vi "RichToFlatmeasurement_StreamRequest.vi"(5 "OutputClusterType":T1, 11 "InputCluster":T2) -> (3 "OutputCluster":T1)   [LabVIEW 2021, in "Measurement_server.lvlib"]
uses:
  Measurement_server.lvlib
  measurement_StreamRequest.ctl
  measurement_StreamRequest_Flat.ctl
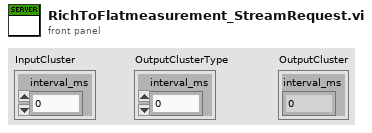
[diagram p1: front panel]
types:
  T1 = typedef "Measurement_server.lvlib/measurement_StreamRequest_Flat.ctl" = cluster{"interval_ms":i32}
  T2 = typedef "Measurement_server.lvlib/measurement_StreamRequest.ctl" = cluster{"interval_ms":i32}
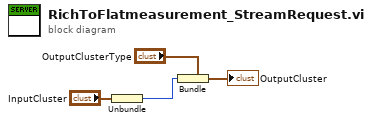
[diagram p0: block diagram]
diagram:
  n1 = Unbundle "Unbundle"("InputCluster") -> ("interval_ms"=w1:i32)
  n2 = Bundle "Bundle"(cluster="OutputClusterType", "interval_ms"=w1) -> (→"OutputCluster":T1)
